vi "IOExpreriments.vi"() -> ()   [LabVIEW 2018]
panel:
  in  "file (use dialog)":path
  in  "Data to be written in the text file":string
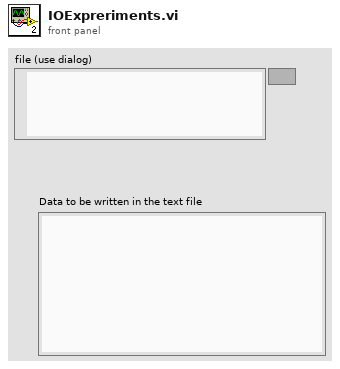
[diagram p1: front panel]
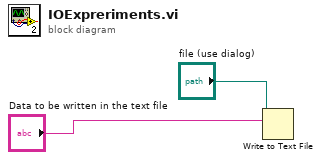
[diagram p0: block diagram]
diagram:
  n1 = Write to Text File(file (use dialog)="file (use dialog)", text="Data to be written in the text file") -> ()  [unwired: 2 in, 3 out]
